vi "Write Scale Multiplier.vi"(8 "error in (no error)":errorcluster, 9 "Index":i32, 10 "Multiplier":dbl, 11 "2D Plot.lvclass in":refnum<class "2D Plot.lvclass">) -> (0 "error out":errorcluster, 3 "2D Plot.lvclass out":refnum<class "2D Plot.lvclass">)   [LabVIEW 2017, in "2D Plot.lvclass"]
uses:
  <vilib>/Math Plots/2D Math Plots/2D Plot/2D Plot/2D Plot.lvclass
  <vilib>/Math Plots/2D Math Plots/2D Plot/2D Plot/2D Plot.lvclass/2D Plot.ctl
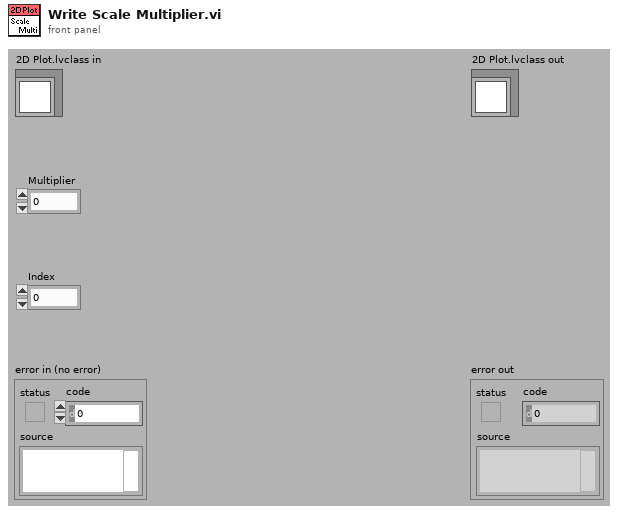
[diagram p1: front panel]
types:
  T1 = typedef "2D Plot.lvclass/Scale Array.ctl" = T2[]
  T2 = typedef "2D Plot.lvclass/Scale Cluster.ctl" = cluster{"General":cluster{"Editable":bool, "Flipped":bool, "Mapping Mode":u8, "Visible":bool, "Style":u8, "Scale Fit":u8}, "Offset and Multiplier":T3, "Range":cluster{"Minimum":dbl, "Maximum":dbl, "Increment":dbl, "Minor Increment":dbl, "Start":dbl}, "Tick Color":cluster{"Major Color":u32, "Minor Color":u32}, "Gird Color":cluster{"Major Color":u32, "Minor Color":u32}, "Marker":cluster{"Visible":bool, "FG Color":u32, "BG Color":u32, "Font Name":string, "Font Size":u32, "Font Bold":bool, "Font Italic":bool, "Font Strikeout":bool, "Font Underline":bool}, "Name Label":cluster{"Visible":bool, "FG Color":u32, "BG Color":u32, "Font Name":string, "Font Size":u32, "Font Bold":bool, "Font Italic":bool, "Font Strikeout":bool, "Font Underline":bool, "Justification":enum16{"Left", "Center", "Right"}, "Text":string}}
  T3 = typedef "LVOffsetAndMultiplierTypeDef.ctl" = cluster{"Offset":dbl, "Multiplier":dbl}
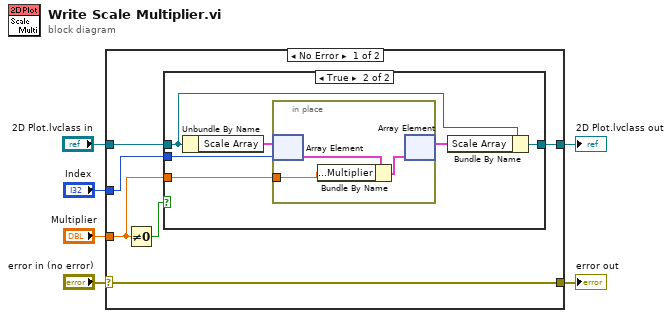
[diagram p0: block diagram]
diagram:
  n1 = case shown="No Error" "error in (no error)" {
    selector: "error in (no error)" -> [w12 w23]
    tunnel: "Multiplier" -> [w7 _]
    tunnel: "2D Plot.lvclass in" -> [w11 w24]
    tunnel: [w10 w24] -> w5
    tunnel: [w12 w23] -> w3
    tunnel: "Index" -> [w9 _]
    frame No Error {
      n2 = Not Equal To 0?(x=w7) -> (x != 0?=w8:bool)
      n3 = case shown="True" w8 {
        tunnel: w11 -> [w13 w19]
        tunnel: [w13 w18] -> w10
        tunnel: w7 -> [_ w16]
        tunnel: w9 -> [_ w14]
        frame False {
        }
        frame True {
          n4 = Unbundle By Name(w19) -> ("Scale Array"=w17:T1)
          n5 = in-place {
            in-place-border: w16 -> [w21]
            n6 = in-place-array #1(w17, w14) -> (w22:T2)
            n7 = Bundle By Name(cluster=w22, "Offset and Multiplier.Multiplier"=w21) -> (w20:T2)
            n8 = in-place-array #1(w20) -> (w15:T1)  [unwired: 1 out]
          }
          n9 = Bundle By Name(cluster=w19, "Scale Array"=w15) -> (w18:refnum<class "2D Plot.lvclass">)
        }
      }
    }
    frame Error {
    }
  }
  "error out" <- w3
  "2D Plot.lvclass out" <- w5
